vi "prueba imaq.vi"() -> ()   [LabVIEW 2010]
uses:
  <vilib>/addons/PixeLINK/Low Level Functions/CAMERA_FEATURES.llb/TDPU-CameraFeatures-PixelFormat.ctl
  <vilib>/addons/PixeLINK/Low Level Functions/CAMERA_FEATURES.llb/TDPU-CameraFeatures-FeatureFlags.ctl
  <vilib>/addons/PixeLINK/Low Level Functions/CAMERA_FEATURES.llb/TDPU-CameraFeatures-FeatureIds.ctl
panel:
  out "Pixel Size (Bytes)":i32
  out "LineWidth(Pixels)":i32
  out "x*y":dbl
  out "Transfer Max Size":i32
  out "Image 2":T1(plugin-control)
  in  "Camera Parameters.Pixel Format":T2 items=["PIXEL_FORMAT_MONO8", "PIXEL_FORMAT_MONO16", "PIXEL_FORMAT_YUV422", "PIXEL_FORMAT_BAYER8_GRBG", "PIXEL_FORMAT_BAYER16_GRBG", "PIXEL_FORMAT_RGB24", "PIXEL_FORMAT_RGB48", "PIXEL_FORMAT_BAYER8_RGGB", "PIXEL_FORMAT_BAYER8_GBRG ", "PIXEL_FORMAT_BAYER8_BGGR ", "PIXEL_FORMAT_BAYER16_RGGB ", "PIXEL_FORMAT_BAYER16_GBRG", "PIXEL_FORMAT_BAYER16_BGGR", "PIXEL_FORMAT_RGB32"]
  out "uBytesPerPixel OUT":u32
  out "uBufferSize OUT":u32
  out "error out":errorcluster
  in  "stop":bool
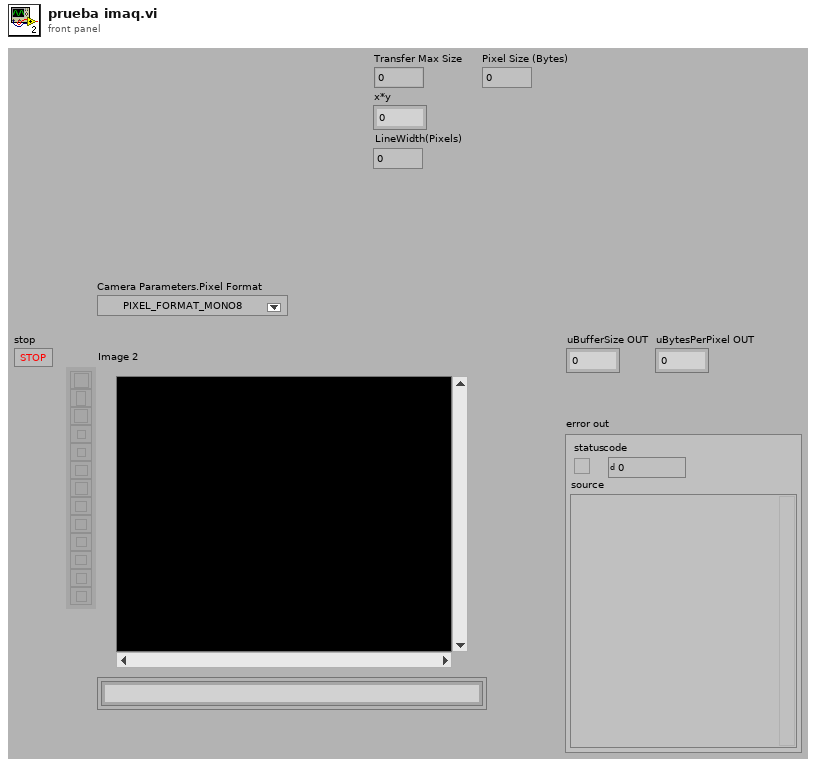
[diagram p1: front panel]
types:
  T1 = typedef "IMAQ Image.ctl" = refnum<image>
  T2 = typedef "TDPU-CameraFeatures-PixelFormat.ctl" = u16
  T3 = typedef "Image Type" = u32
  T4 = typedef "TDPU-CameraFeatures-FeatureFlags.ctl" = u32
  T5 = typedef "TDPU-CameraFeatures-FeatureIds.ctl" = u32
  T6 = cluster{"Exposure Time (ms)":dbl, "Gain (dB)":dbl, "Saturation (%)":dbl, "Brightness (%)":dbl, "Color Temperature":dbl, "ROI":cluster{"Top":i32, "Left":i32, "Width":i32, "Height":i32}, "White Balance Gain (dB)":cluster{"Red":dbl, "Green":dbl, "Blue":dbl}, "Gamma":dbl, "Pixel Format":T2}
  T7 = enum32{"Map Pixel Pointer", "Unmap Pixel Pointer", "Get Pixels Infos"}
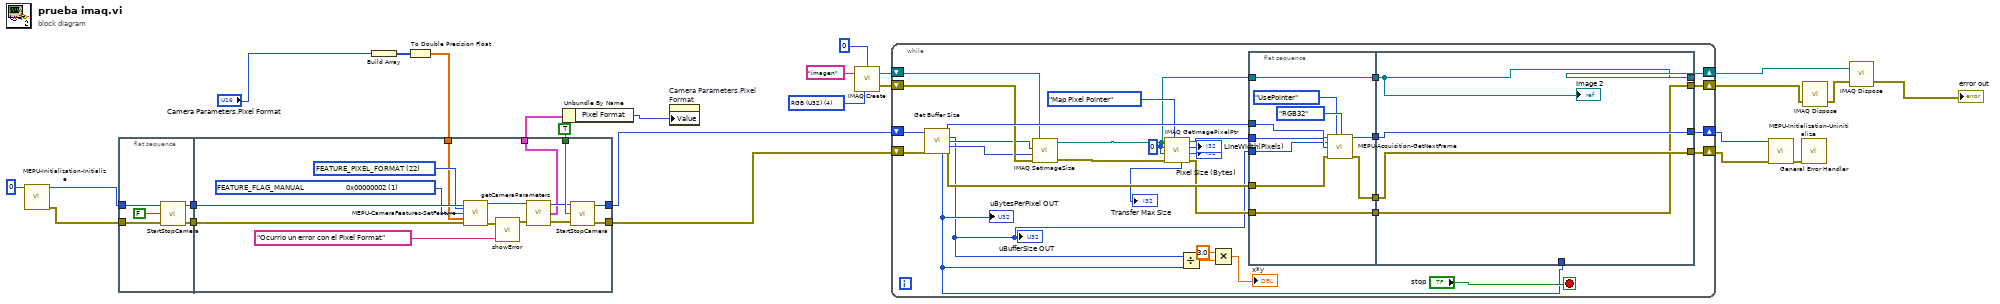
[diagram p0: block diagram]
diagram:
  w23 = T3 4 items=["Grayscale (U8)", "Grayscale (I16)", "Grayscale (SGL)", "Complex (CSG)", "RGB (U32)", "HSL (U32)", "RGB (U64)", "Grayscale (U16)"] ("Image Type")
  n1 = call <vilib>:"MEPU-Initialization-Initialize.vi"("uSerialNumber IN"=u32 0) -> ("phCamera OUT"=w6:u32, "Error OUT"=w7:errorcluster)  [unwired: 1 in, 12 out]
  n2 = flat-sequence {
    tunnel: w6 -> [w29]
    tunnel: w7 -> [w28]
    tunnel: [w27] -> w15
    tunnel: [w26] -> w14
    tunnel: TRUE ("Stream?") -> [w45]
    tunnel: [w44] -> w5
    tunnel: [w43] -> w4
    tunnel: w15 -> [w42]
    tunnel: w14 -> [w41]
    tunnel: [w35] -> w10
    tunnel: w12 -> [w34]
    frame #0 {
      n3 = call "StartStopCamera.vi"("Error IN"=w28, "Camara ON?"=FALSE, "hCamera IN"=w29) -> ("Error OUT"=w26:errorcluster, "hCamera OUT"=w27:u32)  [unwired: 1 in]
    }
    frame #1 {
      w39 = T4 1 items=["FEATURE_FLAG_PRESENCE                 0x00000001", "FEATURE_FLAG_MANUAL                     0x00000002", "FEATURE_FLAG_AUTO                         0x00000004", "FEATURE_FLAG_ONEPUSH                   0x00000008", "FEATURE_FLAG_OFF                            0x00000010", "FEATURE_FLAG_DESC_SUPPORTED    0x00000020", "FEATURE_FLAG_READ_ONLY               0x00000040"] ("uFlags IN")
      w40 = T5 22 items=["FEATURE_BRIGHTNESS", "FEATURE_EXPOSURE", "FEATURE_SHARPNESS", "FEATURE_WHITE_BAL", "FEATURE_HUE", "FEATURE_SATURATION", "FEATURE_GAMMA", "FEATURE_SHUTTER", "FEATURE_GAIN", "FEATURE_IRIS", "FEATURE_FOCUS", "FEATURE_TEMPERATURE", "FEATURE_TRIGGER", "FEATURE_ZOOM", "FEATURE_PAN", "FEATURE_TILT", "FEATURE_OPT_FILTER", "FEATURE_GPIO", "FEATURE_FRAME_RATE", "FEATURE_ROI", "FEATURE_FLIP", "FEATURE_PIXEL_ADDRESSING", "FEATURE_PIXEL_FORMAT", "FEATURE_EXTENDED_SHUTTER", "FEATURE_AUTO_ROI", "FEATURE_LOOKUP_TABLE", "FEATURE_MEMORY_CHANNEL", "FEATURE_WHITE_SHADING", "FEATURE_ROTATE", "FEATURE_IMAGER_CLK_DIVISOR", "FEATURE_TRIG_WITH_CNTRLD_LIGHT", "FEATURE_MAX_PIXEL_SIZE"] ("uFeatureId IN")
      n4 = call <vilib>:"MEPU-CameraFeatures-SetFeature.vi"("hCamera IN"=w42, "uFeatureId IN"=w40, "uFlags IN"=w39, "pParms IN"=w34, "Error IN"=w41) -> ("hCamera OUT"=w38:u32, "Error OUT"=w33:errorcluster)  [unwired: 8 in, 1 out]
      n5 = call "showError.vi"("message"="Ocurrio un error con el Pixel Format", "Error IN"=w33) -> ("Error OUT"=w32:errorcluster)  [unwired: 3 in]
      n6 = call "getCameraParameters.vi"("Error IN"=w32, "hCamera IN"=w38) -> ("Error OUT"=w36:errorcluster, "Camera Parameters"=w35:T6, "hCamera OUT"=w37:u32)  [unwired: 1 in]
      n7 = call "StartStopCamera.vi"("Error IN"=w36, "Camara ON?"=w45, "hCamera IN"=w37) -> ("Error OUT"=w43:errorcluster, "hCamera OUT"=w44:u32)  [unwired: 1 in]
    }
  }
  n8 = Build Array("Camera Parameters.Pixel Format") -> (w13:T2[])
  n9 = To Double Precision Float(number=w13) -> (double precision float=w12:dbl[])
  n10 = Unbundle By Name(w10) -> ("Pixel Format"=w9:T2)
  n11 = property on="Camera Parameters.Pixel Format" class="Ring (strict)"("Value"=w9) -> ()  [unwired: 2 in, 2 out]
  n12 = call "IMAQ Create"("Border Size"=0, "Image Name"="imagen", "Image Type"=w23) -> ("New Image"=w22:T1, "error out"=w21:errorcluster)  [unwired: 2 in]
  n13 = while {
    shift-right: [w68] -> w16
    shift-left: w22 -> [w48]
    shift-right: [w55] -> w2
    shift-left: w21 -> [w71]
    shift-right: [w57] -> w19
    shift-left: w5 -> [w73]
    shift-right: [w56] -> w18
    shift-left: w4 -> [w72]
    stop <- "stop" stop-if-true
    w53 = 0 ("X Coordinate")
    n14 = call "Get Buffer Size.vi"("phCamera IN"=w73, "Error IN"=w72) -> ("phCamera OUT"=w75:u32, "uBufferSize OUT"=w46:u32, "uWidth OUT"=w60:u32, "uHeight OUT"=w59:u32, "uBytesPerPixel OUT"=w58:u32, "Error OUT"=w74:errorcluster)  [unwired: 8 out]
    "uBufferSize OUT" <- w46
    "uBytesPerPixel OUT" <- w58
    n15 = call "IMAQ SetImageSize"("error in (no error)"=w71, "Y Resolution"=w59, "X Resolution"=w60, "Image"=w48) -> ("error out"=w49:errorcluster, "Image Out"=w47:T1)  [unwired: 1 in]
    n16 = call "IMAQ GetImagePixelPtr"("Function"=T7."Map Pixel Pointer", "error in (no error)"=w49, "Y Coordinate"=w53, "X Coordinate"=w53, "Image"=w47) -> ("error out"=w69:errorcluster, "Pixel Size (Bytes)"=→"Pixel Size (Bytes)":i32, "LineWidth(Pixels)"=→"LineWidth(Pixels)":i32, "Pixel Pointer out"=w76:u64, "Transfer Max Size"=→"Transfer Max Size":i32)  [unwired: 1 in, 1 out]
    n17 = Divide(x=w46, y=w58) -> (x/y=w62:dbl)
    n18 = Multiply(x=3.0, y=w62) -> (x*y=→"x*y":dbl)
    n19 = flat-sequence {
      tunnel: w76 -> [w84]
      tunnel: w46 -> [w83]
      tunnel: w74 -> [w82]
      tunnel: w75 -> [w81]
      tunnel: [w80] -> w70
      tunnel: w47 -> [w80]
      tunnel: w69 -> [w79]
      tunnel: [w79] -> w67
      tunnel: [w78] -> w65
      tunnel: [w77] -> w64
      tunnel: w70 -> [w90]
      tunnel: [w90] -> w68
      tunnel: w67 -> [w87]
      tunnel: w65 -> [w89]
      tunnel: w64 -> [w88]
      tunnel: w58 -> [_]
      tunnel: [w89] -> w57
      tunnel: [w88] -> w56
      tunnel: [w87] -> w55
      frame #0 {
        n20 = call <vilib>:"MEPU-Acquisition-GetNextFrame.vi"("hCamera IN"=w81, "Mode IN"=enum16{"UseArray", "UsePointer"}."UsePointer", "OutputMode IN"=enum16{"Default", "RGB24", "RGB32"}."RGB32", "uBufferSize IN"=w83, "pPixel IN"=w84, "Error IN"=w82) -> ("hCamera OUT"=w78:u32, "Error OUT"=w77:errorcluster)  [unwired: 5 in, 3 out]
      }
      frame #1 {
        "Image 2" <- w90
      }
    }
  }
  n21 = call <vilib>:"MEPU-Initialization-Uninitialize.vi"("hCamera IN"=w19, "Error IN"=w18) -> ("Error OUT"=w20:errorcluster)  [unwired: 13 out]
  n22 = call <vilib>:"General Error Handler.vi"("error in (no error)"=w20) -> ()  [unwired: 2 in, 13 out]
  n23 = call "IMAQ Dispose"("error in (no error)"=w2) -> ("error out"=w3:errorcluster)  [unwired: 5 in]
  n24 = call "IMAQ Dispose"("Image"=w16, "error in (no error)"=w3) -> ("error out"=→"error out":errorcluster)  [unwired: 4 in]
